vi "Column Titles--Const.vi"() -> (3 "Column Titles":string[](array[string]))   [LabVIEW 2017, in "Communications Library.lvlib"]
uses:
  Communications Library.lvlib
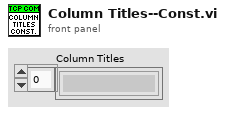
[diagram p1: front panel]
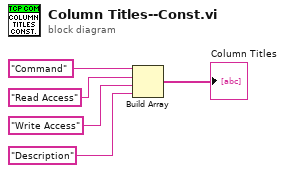
[diagram p0: block diagram]
diagram:
  n1 = Build Array("Command", "Read Access", "Write Access", "Description") -> (→"Column Titles":string[])
